vi "Disable All Outputs.vi"(8 "error in":errorcluster, 11 "DIG_IO in":refnum<class "DIG_IO.lvclass">) -> (0 "error out":errorcluster, 3 "DIG_IO out":refnum<class "DIG_IO.lvclass">)   [LabVIEW 2019]
uses:
  builds/Engine/Engine.lvlibp/Project/Engine.lvclass
  builds/Instruments/Instruments.lvlibp/Library/Instruments.lvclass
  Library/DIG_IO.lvclass
  builds/Instruments/Instruments.lvlibp/Private/Polymorphic/Special/Event from String.vi
  builds/Instruments/Instruments.lvlibp
  C:/Users/Public/Documents/Development/builds/Instruments/Instruments.lvlibp/Library/Instruments.lvclass
  C:/Users/Public/Documents/Development/builds/Tools/Config.lvlibp/Config.lvclass
  C:/Users/Public/Documents/Development/builds/Engine/Engine.lvlibp/Project/Engine.lvclass
  C:/Users/Public/Documents/Development/builds/Engine/Panel Manager.lvlibp/Panel Actor/Panel Actor.lvclass
  C:/Users/Public/Documents/Development/builds/Engine/Monitored Actor.lvlibp/Monitored Actor/Monitored Actor/Monitored Actor.lvclass
  C:/Users/Public/Documents/Development/builds/Engine/Actor Framework.lvlibp/1abvi3w/vi.lib/ActorFramework/Actor/Actor.lvclass
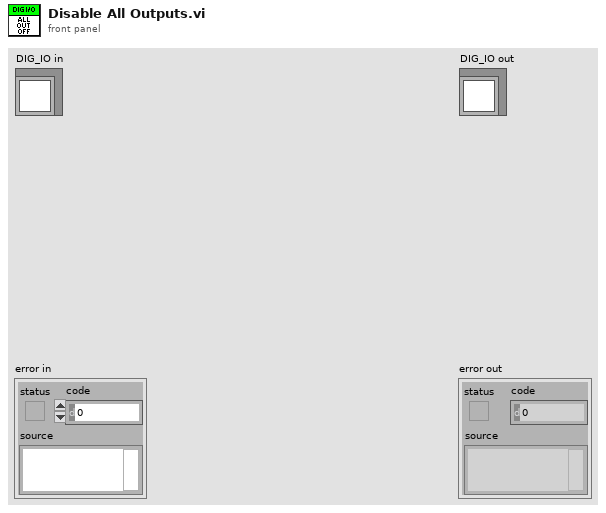
[diagram p1: front panel]
types:
  T1 = cluster{"Timestamp":timestamp, "Description":string, "Data":string}
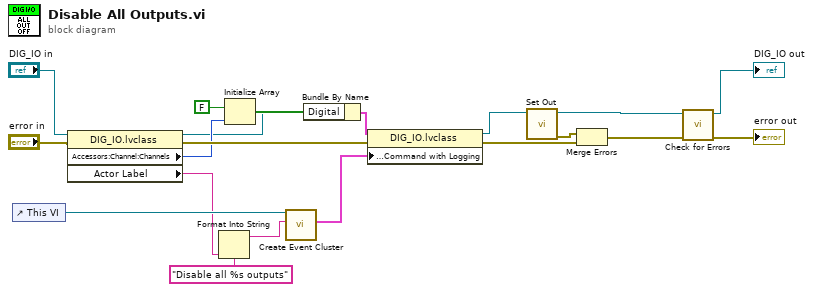
[diagram p0: block diagram]
diagram:
  n1 = control-ref of="This VI"() -> (w9:refnum<vi>)
  n2 = property class="DIG_IO.lvclass"(reference="DIG_IO in", error in="error in") -> (reference out=w4:refnum<class "DIG_IO.lvclass">, error out=w7:errorcluster, "Accessors:Channel:Channels"=w5:u32, "Actor Label"=w1:string)
  n3 = Format Into String(format string="Disable all %s outputs", w1) -> (resulting string=w3:string)  [unwired: 2 in, 1 out]
  n4 = Initialize Array(FALSE, w5) -> (w19:bool[])
  n5 = call-poly "Create Event Cluster.vi"("Value"=w3, "VI Refnum"=w9) -> ("Event Data"=w10:T1)  [unwired: 9 in]
  n6 = Bundle By Name(cluster=w4, "Digital"=w19) -> (w13:cluster{})
  n7 = property class="DIG_IO.lvclass"(reference=w13, error in=w7, "Accessors:Logging:Command with Logging"=w10) -> (reference out=w11:refnum<class "DIG_IO.lvclass">, error out=w12:errorcluster)
  n8 = call-dynamic "Set Out.vi"("DIG_IO in"=w11) -> ("error out"=w18:errorcluster, "DIG_IO out"=w16:refnum<class "DIG_IO.lvclass">)  [unwired: 9 in]
  n9 = Merge Errors(w18, w12) -> (w17:errorcluster)
  n10 = call "Check for Errors.vi"("error in"=w17, "Engine in"=w16) -> ("error out"=→"error out":errorcluster, "Engine out"=→"DIG_IO out":refnum<class "DIG_IO.lvclass">)  [unwired: 8 in]
